vi "PSDs.vi"(0 "X":dbl[](array[numeric]), 1 "averaging done":bool, 5 "Y":dbl[](array[numeric]), 7 "sum":dbl[](array[numeric]), 9 "dt":dbl, 12 "error in (no error)":errorcluster) -> (4 "X":waveform(dbl), 6 "Y":waveform(dbl), 8 "Sum":waveform(dbl), 10 "PSDX":dynamicdata(graph), 13 "error out":errorcluster, 14 "PSDsum":dynamicdata(graph), 15 "PSDY":dynamicdata(graph))   [LabVIEW 2019]
uses:
  <vilib>/express/express analysis/Spectral/Block/exnSpectralBlock spectral measurements PSD poly.vi
  <vilib>/express/express analysis/Spectral/Block/exnSpectralBlock spectral measurements PSD DDT.vi
  <vilib>/express/express analysis/Spectral/XNode/ExpressSpectralMeasurementsBlockNode.xnode
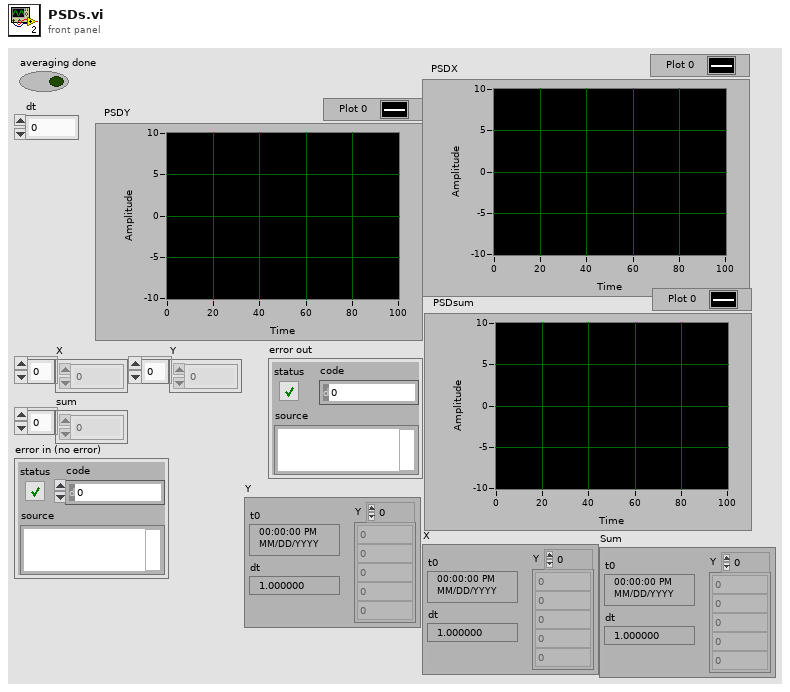
[diagram p1: front panel]
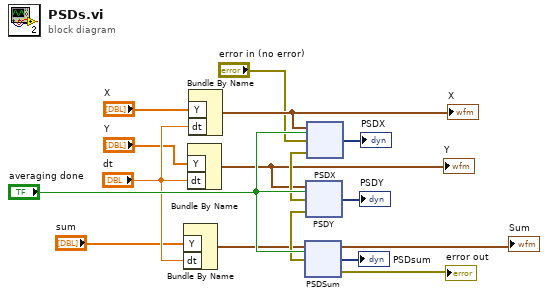
[diagram p0: block diagram]
diagram:
  n1 = Bundle By Name("Y"="sum", "dt"="dt") -> (w3:waveform(dbl))  [unwired: 1 in]
  "Sum" <- w3
  n2 = Bundle By Name("Y"="Y", "dt"="dt") -> (w4:waveform(dbl))  [unwired: 1 in]
  "Y" <- w4
  n3 = Bundle By Name("Y"="X", "dt"="dt") -> (w5:waveform(dbl))  [unwired: 1 in]
  "X" <- w5
  n4 = xnode "PSDX"("Signals"=w5, "Restart Averaging"="averaging done", "error in (no error)"="error in (no error)") -> ("PSD"=→"PSDX":dynamicdata, "error out"=w11:errorcluster)  [unwired: 1 out]
  n5 = xnode "PSDY"("Signals"=w4, "Restart Averaging"="averaging done", "error in (no error)"=w11) -> ("PSD"=→"PSDY":dynamicdata, "error out"=w10:errorcluster)  [unwired: 1 out]
  n6 = xnode "PSDSum"("Signals"=w3, "Restart Averaging"="averaging done", "error in (no error)"=w10) -> ("PSD"=→"PSDsum":dynamicdata, "error out"=→"error out":errorcluster)  [unwired: 1 out]
